vi "CoinDetector.vi"() -> ()   [LabVIEW 2020]
panel:
  out "Waveform Chart 2":dynamicdata(graph)
  in  "number of samples":i32=10
  in  "rate":dbl=2000.0
  out "Waveform Chart":dynamicdata(graph)
  in  "stop":bool
  out "Numeric":dbl
  out "Vpp":dbl
  out "freqency":dbl
  out "Vout":dbl
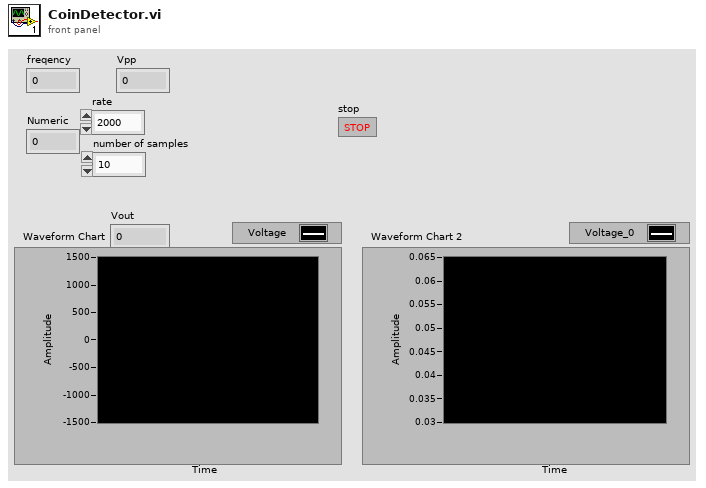
[diagram p1: front panel]
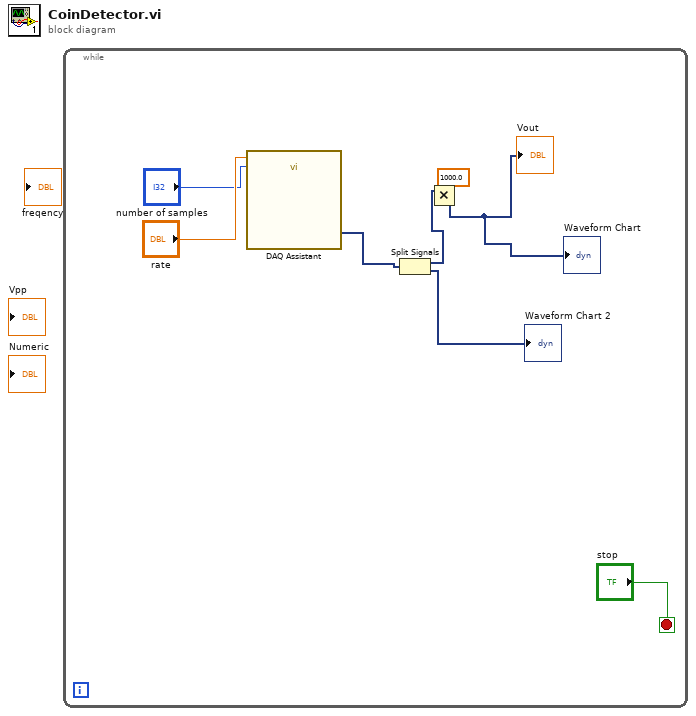
[diagram p0: block diagram]
diagram:
  n1 = while {
    stop <- "stop" stop-if-true
    n2 = call "DAQ Assistant"("rate"="rate", "number of samples"="number of samples") -> ("data"=w3:dynamicdata)  [unwired: 14 in, 3 out]
    n3 = Split Signals(w3) -> (w2:dynamicdata, →"Waveform Chart 2":dynamicdata)  [unwired: 2 in]
    n4 = Multiply(x=w2, y=1000.0) -> (x*y=→"Vout" →"Waveform Chart":dynamicdata)
  }
